vi "Enable Controls.vi"(8 "error in (no error)":errorcluster, 9 "enable":bool=TRUE, 11 "Control":refnum<vi>[](array[refnum])) -> (0 "error out":errorcluster)   [LabVIEW 2018]
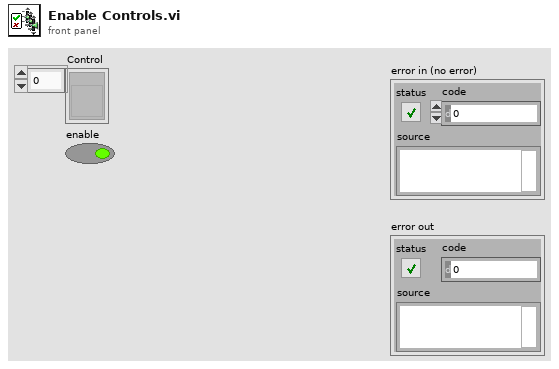
[diagram p1: front panel]
types:
  T1 = enum8{"Enabled", "Disabled", "Disabled and Grayed Out"}
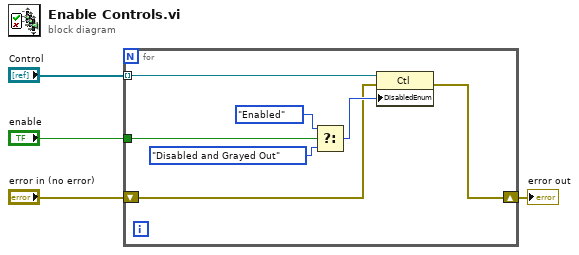
[diagram p0: block diagram]
diagram:
  n1 = for {
    tunnel: "Control" -> [w11] mode=indexing
    tunnel: "enable" -> [w10]
    shift-right: [w5] -> w1
    shift-left: "error in (no error)" -> [w6]
    n2 = Select(t=T1."Enabled" ("Disabled"), s=w10, f=T1."Disabled and Grayed Out" ("Disabled")) -> (s? t:f=w7:T1)
    n3 = property on="Property Node" class="Ctl"(reference=w11, error in=w6, "DisabledEnum"=w7) -> (error out=w5:errorcluster)  [unwired: 1 out]
  }
  "error out" <- w1
